vi "401_Unauthorized_fromNET.vi"(8 "error in (no error)":errorcluster, 11 "headers":string="HTTP/1.1 401 Unauthorized\r\nWWW-Authenticate: Digest realm=\"Login to 4H0572FPAG801C6\", qop=\"auth\", nonce=\"1763322981\", opaque=\"a663b9f7478c0416c2eaa1c598bca2154a0b27af\"\r\nConnection: close\r\nCONTENT-LENGTH: 0\r\n\r\nHTTP/1.1 400 Bad Request\r\nConnection: close\r\nContent-type: text/plain;charset=utf-8\r\nContent-Length: 21\r\n\r\n") -> (0 "error out":errorcluster, 2 "ServerInfo":T1={"realm"="Login to 4H0572FPAG801C6", "qop"="auth", "nounce"="\u0017c2)", "opaque"="a663b9f7478c0416c2eaa1c598bca2154a0b27af"})   [LabVIEW 2016]
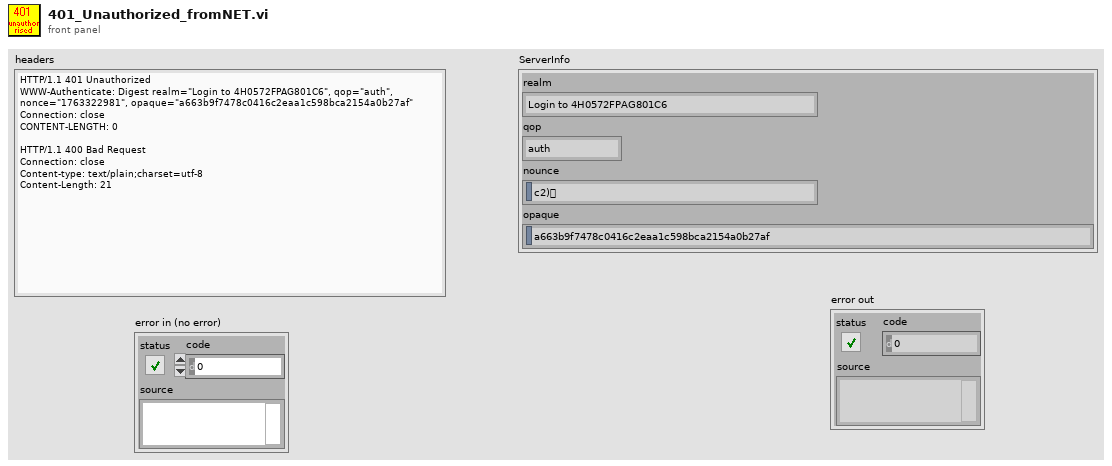
[diagram p1: front panel]
types:
  T1 = cluster{"realm":string, "qop":string, "nounce":string, "opaque":string}
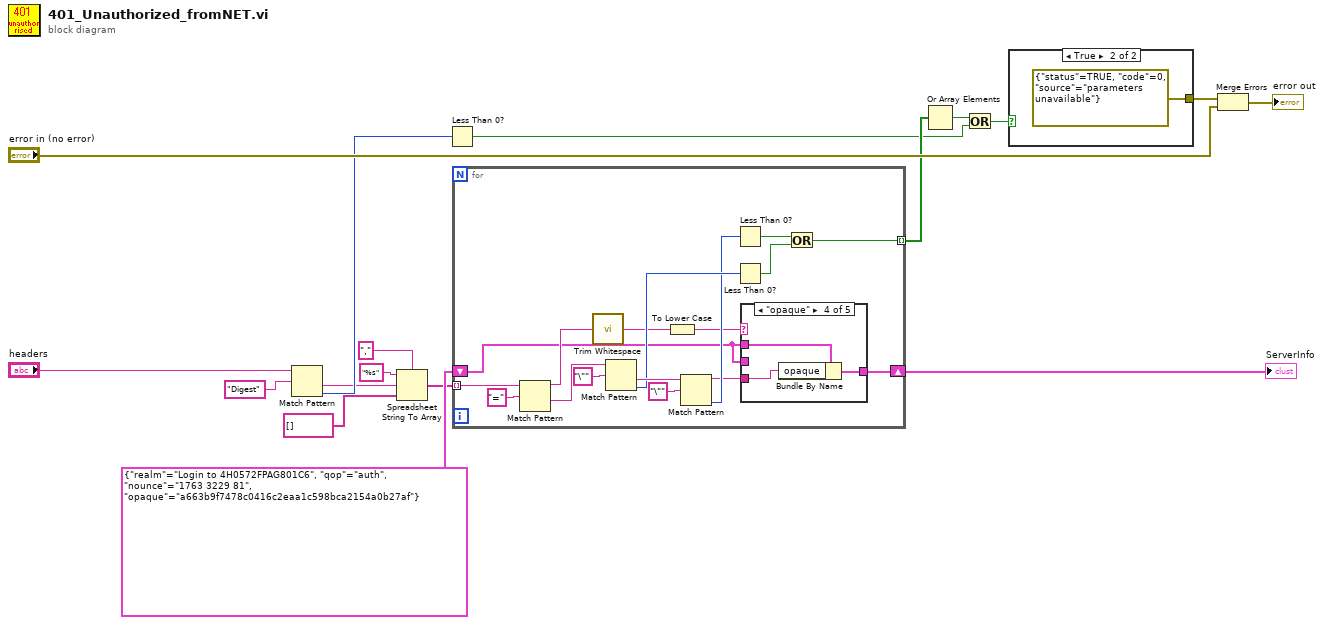
[diagram p0: block diagram]
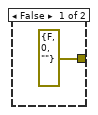
[diagram p2: hidden frame]
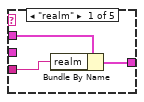
[diagram p3: hidden frame]
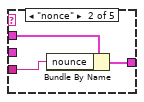
[diagram p4: hidden frame]
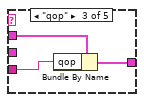
[diagram p5: hidden frame]
diagram:
  n1 = Match Pattern(string="headers", regular expression="Digest") -> (after substring=w1:string, offset past match=w7:i32)  [unwired: 1 in, 2 out]
  n2 = Spreadsheet String To Array(delimiter (Tab)=",", format string="%s", spreadsheet string=w1, array type (2D Dbl)=string[] [] ("Array Constant")) -> (array=w8:string[])
  n3 = Less Than 0?(x=w7) -> (x < 0?=w5:bool)
  n4 = for {
    tunnel: w8 -> [w33] mode=indexing
    tunnel: [w24] -> w6 mode=indexing
    shift-right: [w19] -> w14
    shift-left: T1 {"realm"="Login to 4H0572FPAG801C6", "qop"="auth", "nounce"="1763 3229 81", "opaque"="a663b9f7478c0416c2eaa1c598bca2154a0b27af"} ("ServerInfo") -> [w18]
    n5 = Match Pattern(string=w33, regular expression="=") -> (before substring=w23:string, after substring=w32:string)  [unwired: 1 in, 2 out]
    n6 = call <vilib>:"Trim Whitespace.vi"("string"=w23) -> ("trimmed string"=w22:string)  [unwired: 1 in]
    n7 = Match Pattern(string=w32, regular expression="\"") -> (after substring=w30:string, offset past match=w28:i32)  [unwired: 1 in, 2 out]
    n8 = To Lower Case(string=w22) -> (all lower case string=w21:string)
    n9 = Match Pattern(string=w30, regular expression="\"") -> (before substring=w20:string, offset past match=w27:i32)  [unwired: 1 in, 2 out]
    n10 = Less Than 0?(x=w27) -> (x < 0?=w26:bool)
    n11 = Less Than 0?(x=w28) -> (x < 0?=w25:bool)
    n12 = case shown="\"opaque\"" w21 {
      tunnel: w18 -> [w37 w40 w43 w46 _]
      tunnel: w20 -> [w35 w39 w42 w45 _]
      tunnel: [w36 w38 w41 w44 w47] -> w19
      tunnel: w18 -> [_ _ _ _ w47]
      frame "realm" {
        n13 = Bundle By Name(cluster=w37, "realm"=w35) -> (w36:T1)
      }
      frame "nonce" {
        n14 = Bundle By Name(cluster=w40, "nounce"=w39) -> (w38:T1)
      }
      frame "qop" {
        n15 = Bundle By Name(cluster=w43, "qop"=w42) -> (w41:T1)
      }
      frame "opaque" {
        n16 = Bundle By Name(cluster=w46, "opaque"=w45) -> (w44:T1)
      }
      frame Default {
      }
    }
    n17 = Or(x=w26, y=w25) -> (x .or. y?=w24:bool)
  }
  "ServerInfo" <- w14
  n18 = Or Array Elements(Boolean array=w6) -> (logical OR=w4:bool)
  n19 = Or(x=w4, y=w5) -> (x .or. y?=w3:bool)
  n20 = case shown="True" w3 {
    tunnel: [errorcluster {"status"=FALSE, "code"=0, "source"=""} ("error constant") errorcluster {"status"=TRUE, "code"=0, "source"="parameters unavailable"} ("error constant")] -> w2
    frame False {
    }
    frame True {
    }
  }
  n21 = Merge Errors(w2, "error in (no error)") -> (→"error out":errorcluster)
